vi "image operation.vi"() -> ()   [LabVIEW 2016]
uses:
  <vilib>/Utility/file.llb/Write Delimited Spreadsheet (I64).vi
  <vilib>/vision/NI_Vision_Development_Module.lvlib
panel:
  out "x*y":i32
  in  "txt-dimension":enum16{"x", "1d", "2d"}(ring)
  in  "X Resolution":i32
  in  "Y Resolution":i32
  in  "File Path 6":path=path "C:/Users/NB-SH-001/Pictures/Calibration Model Accuracy - Parts/Part 18.jpg"
  in  "File Path 5":path=path "C:/Users/NB-SH-001/Pictures/Calibration Model Accuracy - Parts/Part 12.jpg"
  out "Image 4":T1(plugin-control)
  out "Image 1":T1(plugin-control)
  out "Image Pixels (U8) 2":u8[][](array[numeric])
  in  "file path":path=path "C:/Users/NB-SH-001/Pictures/test_img/1/1-1_1392x1040_18.txt" caption="파일 경로(비었을 경우 대화 상자 창)"
  in  "operation":enum16{"and", "xor", "or", "add"}(ring)
  in  "File Path 4":path=path "C:/Users/NB-SH-001/Pictures/Calibration Model Accuracy - Parts/Part 06.jpg"
  in  "img-N":u8=1
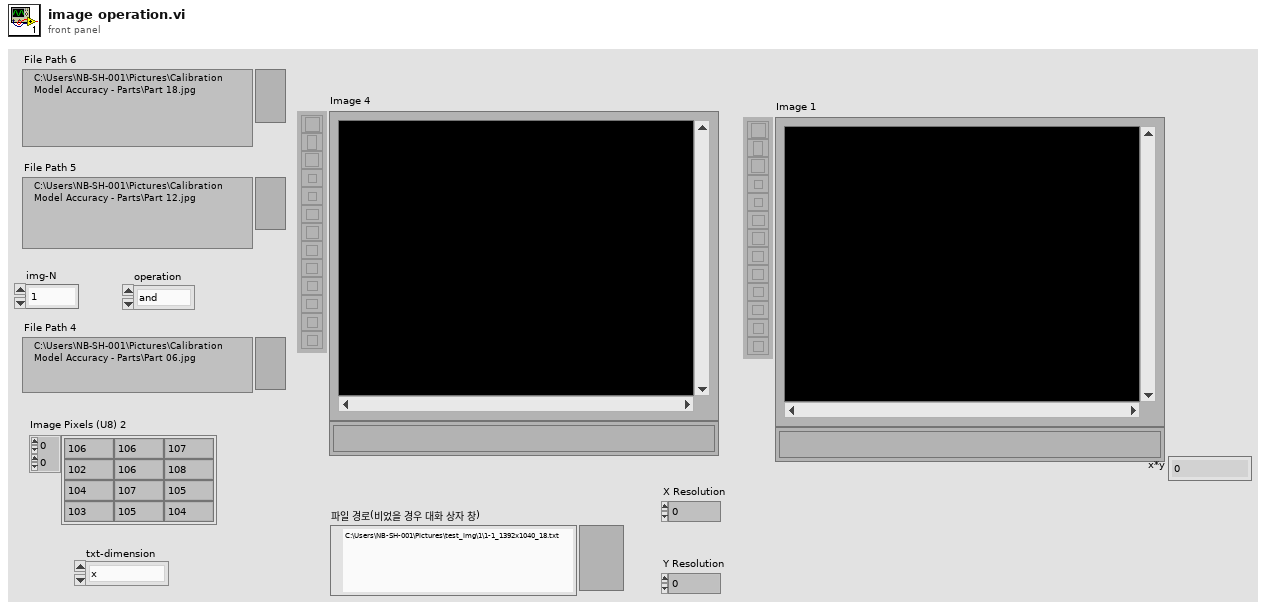
[diagram p1: front panel]
types:
  T1 = typedef "IMAQ Image.ctl" = refnum<image>
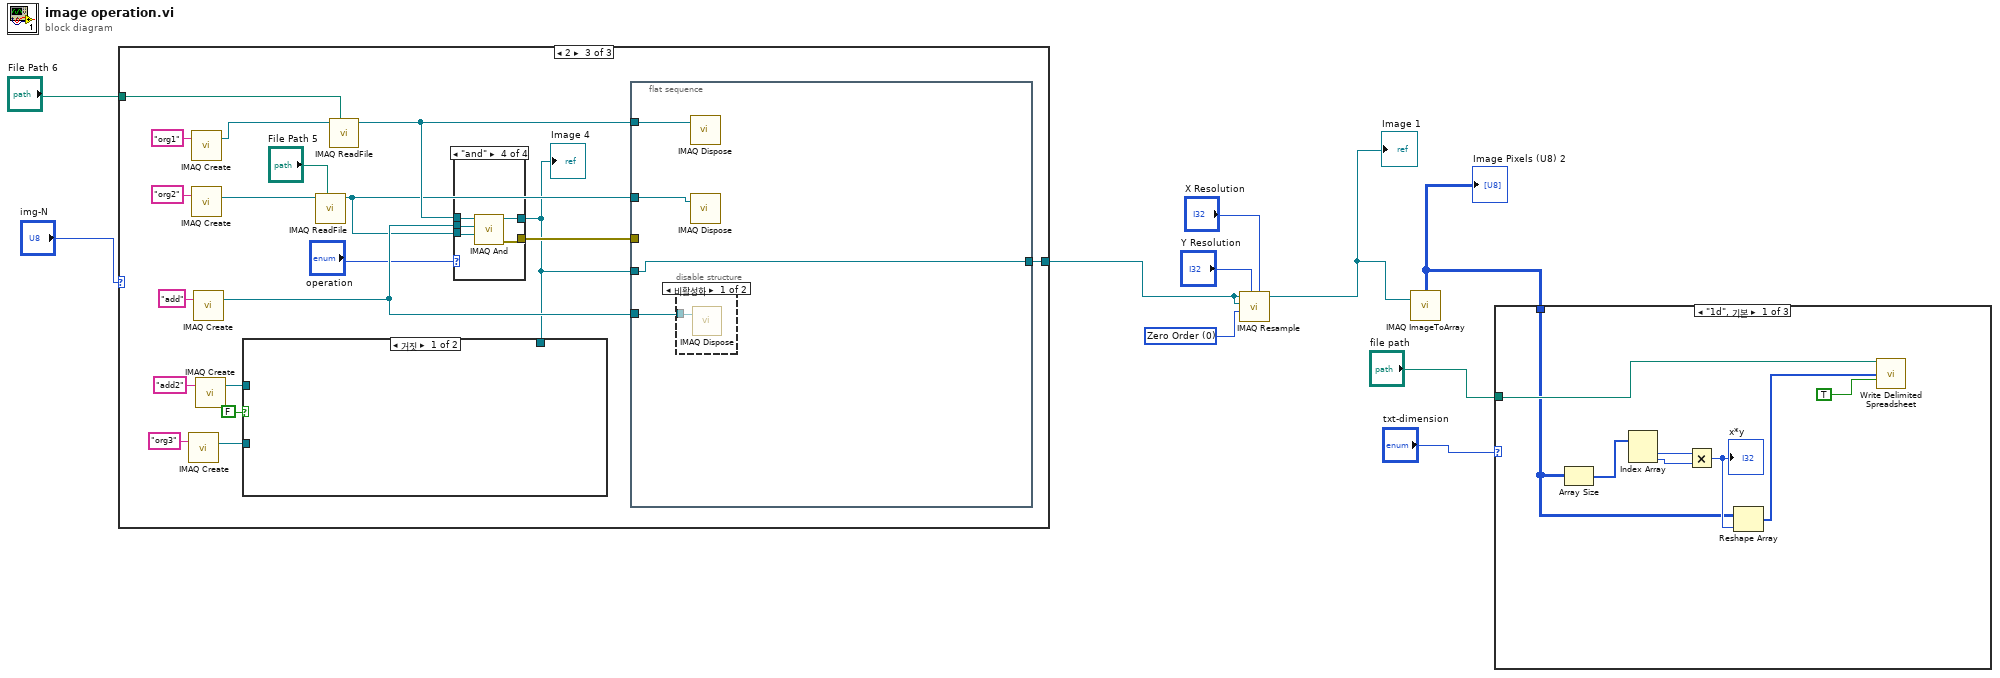
[diagram p0: block diagram]
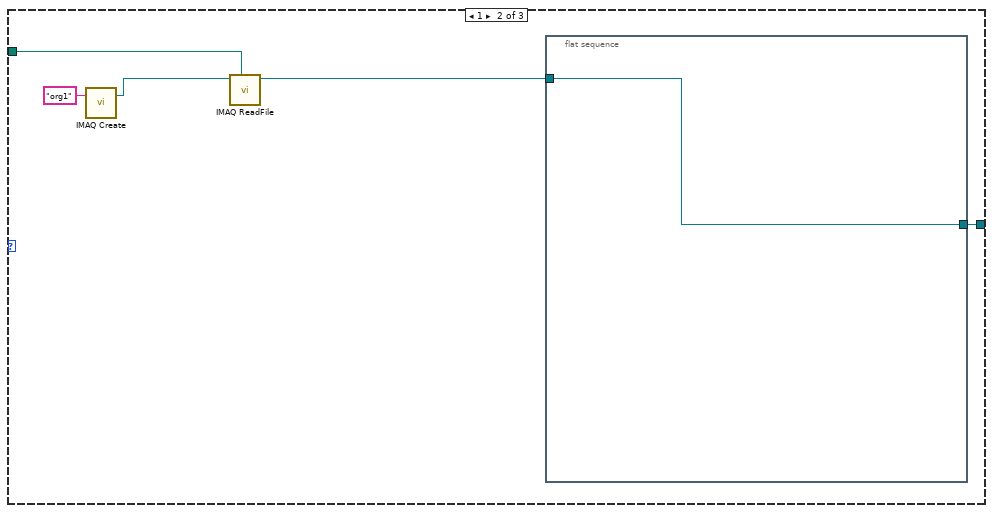
[diagram p5: hidden frame]
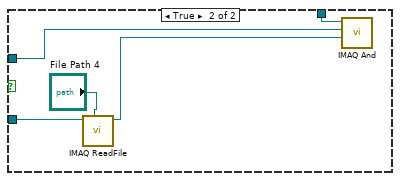
[diagram p6: hidden frame]
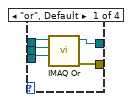
[diagram p7: hidden frame]
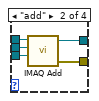
[diagram p8: hidden frame]
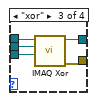
[diagram p9: hidden frame]
diagram:
  w1 = u32 0 items=["Zero Order", "Bi-Linear", "Quadratic", "Cubic Spline"] ("Interpolation Type")
  n1 = case shown="2" "img-N" {
    tunnel: [_ w13 w19] -> w3
    tunnel: "File Path 6" -> [_ w12 w18]
    frame 0, Default {
    }
    frame 1 {
      n2 = call "IMAQ Create"("Image Name"="org1") -> ("New Image"=w14:T1)  [unwired: 4 in, 1 out]
      n3 = call "IMAQ ReadFile"("File Path"=w12, "Image"=w14) -> ("Image Out"=w11:T1)  [unwired: 5 in, 4 out]
      n4 = flat-sequence {
        tunnel: w11 -> [w16]
        tunnel: [w16] -> w13
        frame #0 {
        }
      }
    }
    frame 2 {
      n5 = call "IMAQ Create"("Image Name"="org3") -> ("New Image"=w22:T1)  [unwired: 4 in, 1 out]
      n6 = call "IMAQ Create"("Image Name"="org1") -> ("New Image"=w32:T1)  [unwired: 4 in, 1 out]
      n7 = call "IMAQ Create"("Image Name"="org2") -> ("New Image"=w31:T1)  [unwired: 4 in, 1 out]
      n8 = call "IMAQ Create"("Image Name"="add") -> ("New Image"=w28:T1)  [unwired: 4 in, 1 out]
      n9 = call "IMAQ Create"("Image Name"="add2") -> ("New Image"=w23:T1)  [unwired: 4 in, 1 out]
      n10 = call "IMAQ ReadFile"("File Path"="File Path 5", "Image"=w31) -> ("Image Out"=w27:T1)  [unwired: 5 in, 4 out]
      n11 = call "IMAQ ReadFile"("File Path"=w18, "Image"=w32) -> ("Image Out"=w29:T1)  [unwired: 5 in, 4 out]
      n12 = case shown="\"and\"" "operation" {
        tunnel: [w42 w50 w55 w60] -> w20
        tunnel: w29 -> [w43 w49 w52 w57]
        tunnel: w28 -> [w44 w48 w53 w58]
        tunnel: w27 -> [w45 w47 w54 w59]
        tunnel: [w41 w46 w51 w56] -> w26
        frame "or", Default {
          n13 = call "IMAQ Or"("Image Src B"=w45, "Image Dst"=w44, "Image Src A"=w43) -> ("error out"=w41:errorcluster, "Image Dst Out"=w42:T1)  [unwired: 7 in]
        }
        frame "add" {
          n14 = call "IMAQ Add"("Image Src A"=w49, "Image Dst"=w48, "Image Src B"=w47) -> ("Image Dst Out"=w50:T1, "error out"=w46:errorcluster)  [unwired: 4 in]
        }
        frame "xor" {
          n15 = call "IMAQ Xor"("Image Src B"=w54, "Image Dst"=w53, "Image Src A"=w52) -> ("error out"=w51:errorcluster, "Image Dst Out"=w55:T1)  [unwired: 7 in]
        }
        frame "and" {
          n16 = call "IMAQ And"("Image Src B"=w59, "Image Dst"=w58, "Image Src A"=w57) -> ("error out"=w56:errorcluster, "Image Dst Out"=w60:T1)  [unwired: 7 in]
        }
      }
      "Image 4" <- w20
      n17 = case shown="거짓" FALSE {
        tunnel: w23 -> [_ w40]
        tunnel: w22 -> [_ w39]
        tunnel: w20 -> [_ w36]
        frame False {
        }
        frame True {
          n18 = call "IMAQ ReadFile"("File Path"="File Path 4", "Image"=w39) -> ("Image Out"=w37:T1)  [unwired: 5 in, 4 out]
          n19 = call "IMAQ And"("Image Src B"=w37, "Image Dst"=w40, "Image Src A"=w36) -> ()  [unwired: 7 in, 2 out]
        }
      }
      n20 = flat-sequence {
        tunnel: w29 -> [w64]
        tunnel: w28 -> [w63]
        tunnel: w27 -> [w62]
        tunnel: w26 -> [_]
        tunnel: w20 -> [w61]
        tunnel: [w61] -> w19
        frame #0 {
          n21 = disable-structure shown="비활성화" {
            disable-tunnel: w63 -> [w65 _]
            frame Disabled {
              n22 = call "IMAQ Dispose"("Image"=w65) -> ()  [unwired: 5 in, 1 out]
            }
            frame Enabled {
            }
          }
          n23 = call "IMAQ Dispose"("Image"=w64) -> ()  [unwired: 5 in, 1 out]
          n24 = call "IMAQ Dispose"("Image"=w62) -> ()  [unwired: 5 in, 1 out]
        }
      }
    }
  }
  n25 = call "IMAQ Resample"("X Resolution"="X Resolution", "Y Resolution"="Y Resolution", "Interpolation Type"=w1, "Image Dst"=w3, "Image Src"=w3) -> ("Image Dst Out"=w2:T1)  [unwired: 5 in, 1 out]
  "Image 1" <- w2
  n26 = call "IMAQ ImageToArray"("Image"=w2) -> ("Image Pixels (U8)"=w8:u8[][])  [unwired: 3 in, 4 out]
  "Image Pixels (U8) 2" <- w8
  n27 = case shown="\"1d\", 기본" "txt-dimension" {
    tunnel: "file path" -> [w73 _ _]
    tunnel: w8 -> [w68 _ _]
    frame "1d", Default {
      n28 = Array Size(array=w68) -> (size(s)=w70:i32[])
      n29 = Index Array(array=w70) -> (element #1=w72:i32, element #2=w71:i32)  [unwired: 2 in]
      n30 = Multiply(x=w72, y=w71) -> (x*y=w69:i32)
      "x*y" <- w69
      n31 = Reshape Array(w68, w69) -> (w67:u8[])
      n32 = call-poly <vilib>:"Write Delimited Spreadsheet.vi"("file path (dialog if empty)"=w73, "1D data"=w67, "append to file? (new file:F)"=TRUE) -> ()  [unwired: 11 in, 2 out]
    }
    frame "2d" {
    }
    frame "x" {
    }
  }
